vi "Write number_of_tactics.vi"(8 "error in (no error)":errorcluster, 10 "number_of_tactics":dbl=4.0, 11 "TableFinalizerRole in":refnum<class "TableFinalizerRole.lvclass">) -> (0 "error out":errorcluster, 3 "TableFinalizerRole out":refnum<class "TableFinalizerRole.lvclass">)   [LabVIEW 2023, in "TableFinalizerRole.lvclass"]
uses:
  TableFinalizerRole.lvclass
  TableFinalizerRole.lvclass/TableFinalizerRole.ctl
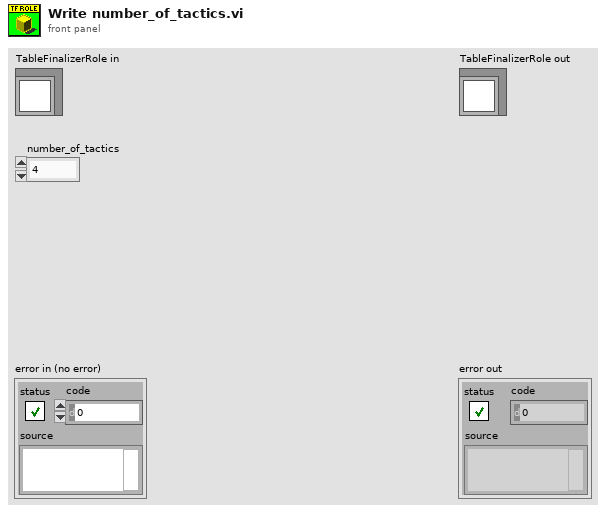
[diagram p1: front panel]
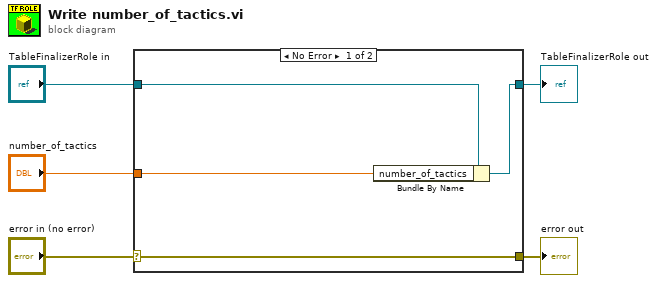
[diagram p0: block diagram]
diagram:
  n1 = case shown="No Error" "error in (no error)" {
    selector: "error in (no error)" -> [w9 w10]
    tunnel: [w9 w10] -> w4
    tunnel: [w7 w11] -> w2
    tunnel: "TableFinalizerRole in" -> [w8 w11]
    tunnel: "number_of_tactics" -> [w6 _]
    frame No Error {
      n2 = Bundle By Name(cluster=w8, "number_of_tactics"=w6) -> (w7:refnum<class "TableFinalizerRole.lvclass">)
    }
    frame Error {
    }
  }
  "error out" <- w4
  "TableFinalizerRole out" <- w2
